vi "GT_SetExtIoValue.vi"(3 "Value":bool, 4 "index":i32, 5 "mdl":i32, 6 "rtn_In":cluster{"rtn":i16, "Func":string}) -> (2 "rtn_Out":cluster{"rtn":i16, "Func":string})   [LabVIEW 2014]
uses:
  data/data/ExtMdl.dll
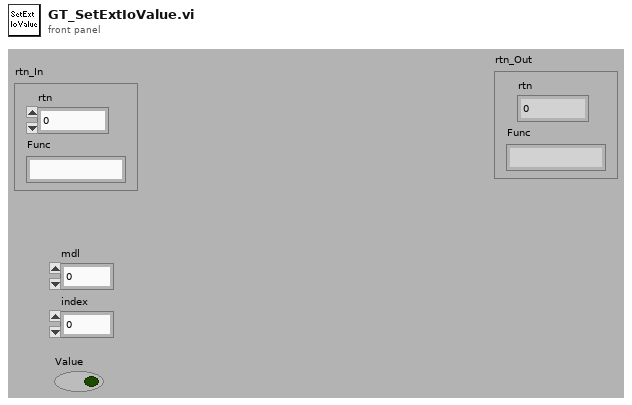
[diagram p1: front panel]
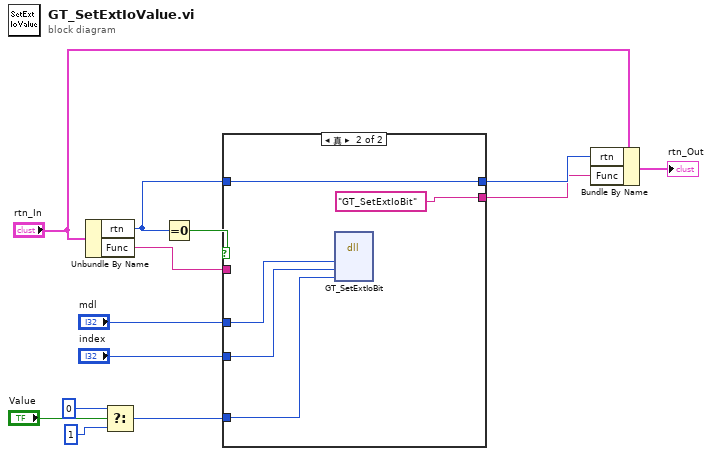
[diagram p0: block diagram]
diagram:
  n1 = Unbundle By Name("rtn_In") -> ("rtn"=w12:i16, "Func"=w8:string)
  n2 = Select(t=0, s="Value", f=1) -> (s? t:f=w1:i32)
  n3 = Equal To 0?(x=w12) -> (x = 0?=w13:bool)
  n4 = case shown="真" w13 {
    tunnel: [w14 w20] -> w11
    tunnel: w12 -> [w14 w20]
    tunnel: [w15 "GT_SetExtIoBit" ("Func")] -> w9
    tunnel: w8 -> [w15 _]
    tunnel: "mdl" -> [_ w18]
    tunnel: "index" -> [_ w17]
    tunnel: w1 -> [_ w16]
    frame False {
    }
    frame True {
      n5 = dll-call lib="PTH2Sabs E\nSourceData&AC-800LWin7标准版源程序-20170923datadata\nExtMdl.dll" fn="GT_SetExtIoBit"("mdl"=w18, "index"=w17, "value"=w16) -> ()  [unwired: 7 in, 2 out]
    }
  }
  n6 = Bundle By Name(cluster="rtn_In", "rtn"=w11, "Func"=w9) -> (→"rtn_Out":cluster{"rtn":i16, "Func":string})
